vi "Loop Period.vi"(1 "Tick Count (Ticks)":u32 caption="时钟计数（滴答）") -> (0 "Loop Period (Ticks)":u32 caption="循环周期（滴答）")   [LabVIEW 2013]
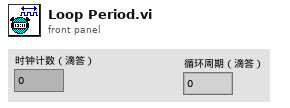
[diagram p1: front panel]
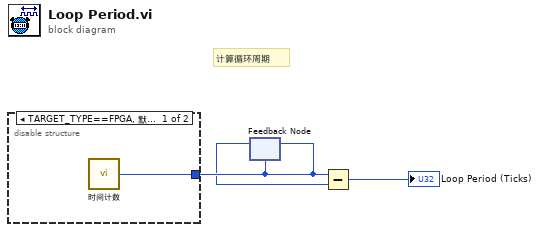
[diagram p0: block diagram]
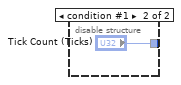
[diagram p2: hidden frame]
diagram:
  # "计算循环周期"
  n1 = disable-structure shown="TARGET_TYPE==FPGA, 默认" {
    disable-tunnel: [w4 "Tick Count (Ticks)"] -> w3
    frame condition #0 (active) {
      n2 = call "时间计数"() -> ("Tick Count(Ticks)"=w4:u32)
    }
    frame condition #1 {
    }
  }
  n3 = feedback #1(w3) -> (w2:u32)
  n4 = feedback-in #1(w3) -> ()
  n5 = Subtract(x=w3, y=w2) -> (x-y=→"Loop Period (Ticks)":u32)
